vi "Trio - Connect.vi"(9 "TrioData In":T1 {"A Axis Parameters"."VPSPEED" format="%#_4g"; "A Axis Parameters"."AXISSTATUS" format="%#_4g"; "A Axis Parameters"."FE" format="%#_4g"; "A Axis Parameters"."MPOS" format="%#_4g"; "A Axis Parameters"."NTYPE" format="%#_4g"; "A Axis Parameters"."MTYPE" format="%#_4g"; "A Axis Parameters"."RS_LIMIT" format="%#_4g"; "A Axis Parameters"."FS_LIMIT" format="%#_4g"; "A Axis Parameters"."FH_IN" format="%#_4g"; "A Axis Parameters"."DATUM_IN" format="%#_4g"; "A Axis Parameters"."REV_IN" format="%#_4g"; "A Axis Parameters"."FWD_IN" format="%#_4g"; "A Axis Parameters"."REP_DIST" format="%#_4g"; "A Axis Parameters"."SERVO" format="%#_4g"; "A Axis Parameters"."DAC" format="%#_4g"; "A Axis Parameters"."FE_LIMIT" format="%#_4g"; "A Axis Parameters"."JOGSPEED" format="%#_4g"; "A Axis Parameters"."CREEP" format="%#_4g"; "A Axis Parameters"."DECEL" format="%#_4g"; "A Axis Parameters"."ACCEL" format="%#_4g"; "A Axis Parameters"."SPEED" format="%#_4g"; "A Axis Parameters"."UNITS" format="%#_4g"; "A Axis Parameters"."VFF_GAIN" format="%#_4g"; "A Axis Parameters"."0V_GAIN" format="%#_4g"; "A Axis Parameters"."D_GAIN" format="%#_4g"; "A Axis Parameters"."I_GAIN" format="%#_4g"; "A Axis Parameters"."P_GAIN" format="%#_4g"; "A Axis Parameters"."ATYPE" format="%#_4g"; "X Axis Parameters"."VPSPEED" format="%#_4g"; "X Axis Parameters"."AXISSTATUS" format="%#_4g"; "X Axis Parameters"."FE" format="%#_4g"; "X Axis Parameters"."MPOS" format="%#_4g"; "X Axis Parameters"."NTYPE" format="%#_4g"; "X Axis Parameters"."MTYPE" format="%#_4g"; "X Axis Parameters"."RS_LIMIT" format="%#_4g"; "X Axis Parameters"."FS_LIMIT" format="%#_4g"; "X Axis Parameters"."FH_IN" format="%#_4g"; "X Axis Parameters"."DATUM_IN" format="%#_4g"; "X Axis Parameters"."REV_IN" format="%#_4g"; "X Axis Parameters"."FWD_IN" format="%#_4g"; "X Axis Parameters"."REP_DIST" format="%#_4g"; "X Axis Parameters"."SERVO" format="%#_4g"; "X Axis Parameters"."DAC" format="%#_4g"; "X Axis Parameters"."FE_LIMIT" format="%#_4g"; "X Axis Parameters"."JOGSPEED" format="%#_4g"; "X Axis Parameters"."CREEP" format="%#_4g"; "X Axis Parameters"."DECEL" format="%#_4g"; "X Axis Parameters"."ACCEL" format="%#_4g"; "X Axis Parameters"."SPEED" format="%#_4g"; "X Axis Parameters"."UNITS" format="%#_4g"; "X Axis Parameters"."VFF_GAIN" format="%#_4g"; "X Axis Parameters"."0V_GAIN" format="%#_4g"; "X Axis Parameters"."D_GAIN" format="%#_4g"; "X Axis Parameters"."I_GAIN" format="%#_4g"; "X Axis Parameters"."P_GAIN" format="%#_4g"; "X Axis Parameters"."ATYPE" format="%#_4g"}, 10 "error in (no error)":errorcluster, 11 "Trio Reference In":refnum<k7>) -> (1 "TrioData Out":T1 {"A Axis Parameters"."VPSPEED" format="%#_4g"; "A Axis Parameters"."AXISSTATUS" format="%#_4g"; "A Axis Parameters"."FE" format="%#_4g"; "A Axis Parameters"."MPOS" format="%#_4g"; "A Axis Parameters"."NTYPE" format="%#_4g"; "A Axis Parameters"."MTYPE" format="%#_4g"; "A Axis Parameters"."RS_LIMIT" format="%#_4g"; "A Axis Parameters"."FS_LIMIT" format="%#_4g"; "A Axis Parameters"."FH_IN" format="%#_4g"; "A Axis Parameters"."DATUM_IN" format="%#_4g"; "A Axis Parameters"."REV_IN" format="%#_4g"; "A Axis Parameters"."FWD_IN" format="%#_4g"; "A Axis Parameters"."REP_DIST" format="%#_4g"; "A Axis Parameters"."SERVO" format="%#_4g"; "A Axis Parameters"."DAC" format="%#_4g"; "A Axis Parameters"."FE_LIMIT" format="%#_4g"; "A Axis Parameters"."JOGSPEED" format="%#_4g"; "A Axis Parameters"."CREEP" format="%#_4g"; "A Axis Parameters"."DECEL" format="%#_4g"; "A Axis Parameters"."ACCEL" format="%#_4g"; "A Axis Parameters"."SPEED" format="%#_4g"; "A Axis Parameters"."UNITS" format="%#_4g"; "A Axis Parameters"."VFF_GAIN" format="%#_4g"; "A Axis Parameters"."0V_GAIN" format="%#_4g"; "A Axis Parameters"."D_GAIN" format="%#_4g"; "A Axis Parameters"."I_GAIN" format="%#_4g"; "A Axis Parameters"."P_GAIN" format="%#_4g"; "A Axis Parameters"."ATYPE" format="%#_4g"; "X Axis Parameters"."VPSPEED" format="%#_4g"; "X Axis Parameters"."AXISSTATUS" format="%#_4g"; "X Axis Parameters"."FE" format="%#_4g"; "X Axis Parameters"."MPOS" format="%#_4g"; "X Axis Parameters"."NTYPE" format="%#_4g"; "X Axis Parameters"."MTYPE" format="%#_4g"; "X Axis Parameters"."RS_LIMIT" format="%#_4g"; "X Axis Parameters"."FS_LIMIT" format="%#_4g"; "X Axis Parameters"."FH_IN" format="%#_4g"; "X Axis Parameters"."DATUM_IN" format="%#_4g"; "X Axis Parameters"."REV_IN" format="%#_4g"; "X Axis Parameters"."FWD_IN" format="%#_4g"; "X Axis Parameters"."REP_DIST" format="%#_4g"; "X Axis Parameters"."SERVO" format="%#_4g"; "X Axis Parameters"."DAC" format="%#_4g"; "X Axis Parameters"."FE_LIMIT" format="%#_4g"; "X Axis Parameters"."JOGSPEED" format="%#_4g"; "X Axis Parameters"."CREEP" format="%#_4g"; "X Axis Parameters"."DECEL" format="%#_4g"; "X Axis Parameters"."ACCEL" format="%#_4g"; "X Axis Parameters"."SPEED" format="%#_4g"; "X Axis Parameters"."UNITS" format="%#_4g"; "X Axis Parameters"."VFF_GAIN" format="%#_4g"; "X Axis Parameters"."0V_GAIN" format="%#_4g"; "X Axis Parameters"."D_GAIN" format="%#_4g"; "X Axis Parameters"."I_GAIN" format="%#_4g"; "X Axis Parameters"."P_GAIN" format="%#_4g"; "X Axis Parameters"."ATYPE" format="%#_4g"}, 2 "error out":errorcluster, 3 "Trio Reference Out":refnum<k7>)   [LabVIEW 2020, in "TrioMotion Controller.lvlib"]
uses:
  TrioMotion Controller.lvlib
  TrioData.ctl
  Connection Type.ctl
  Axis Parameters.ctl
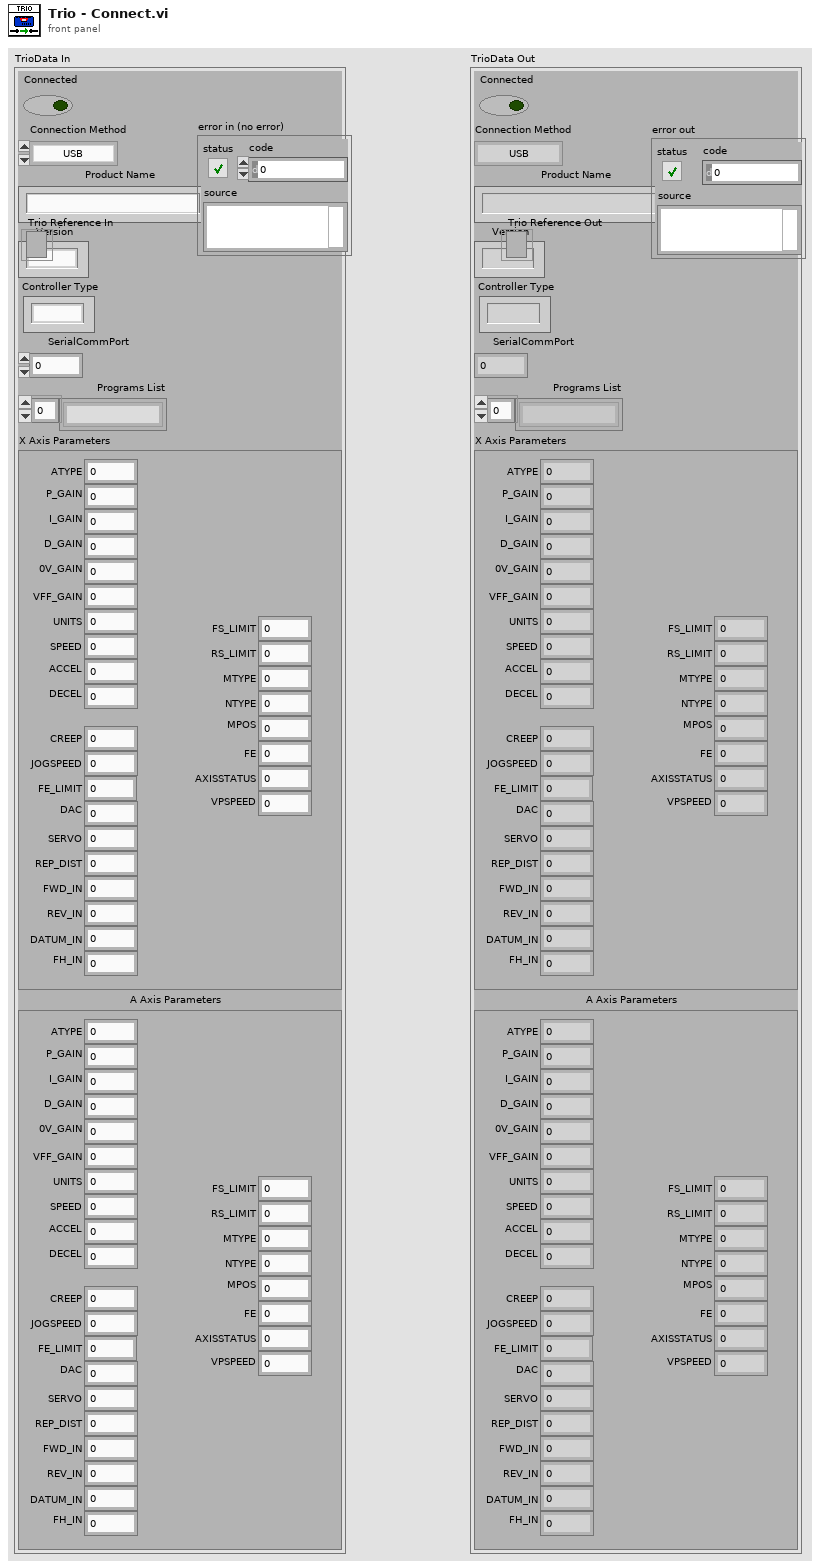
[diagram p1: front panel]
types:
  T1 = typedef "TrioMotion Controller.lvlib/TrioData.ctl" = cluster{"Connected":bool, "Connection Method":T2, "Product Name":string, " Version":string, "Controller Type":string, "SerialCommPort":fxp<+,3,3>, "Programs List":string[], "X Axis Parameters":T3, "A Axis Parameters":T3}
  T2 = typedef "TrioMotion Controller.lvlib/Connection Type.ctl" = enum16{"USB", "Serial", "Ethernet", "PCI", "Path", "No connection"}
  T3 = typedef "TrioMotion Controller.lvlib/Axis Parameters.ctl" = cluster{"ATYPE":dbl, "P_GAIN":dbl, "I_GAIN":dbl, "D_GAIN":dbl, "0V_GAIN":dbl, "VFF_GAIN":dbl, "UNITS":dbl, "SPEED":dbl, "ACCEL":dbl, "DECEL":dbl, "CREEP":dbl, "JOGSPEED":dbl, "FE_LIMIT":dbl, "DAC":dbl, "SERVO":dbl, "REP_DIST":dbl, "FWD_IN":dbl, "REV_IN":dbl, "DATUM_IN":dbl, "FH_IN":dbl, "FS_LIMIT":dbl, "RS_LIMIT":dbl, "MTYPE":dbl, "NTYPE":dbl, "MPOS":dbl, "FE":dbl, "AXISSTATUS":dbl, "VPSPEED":dbl}
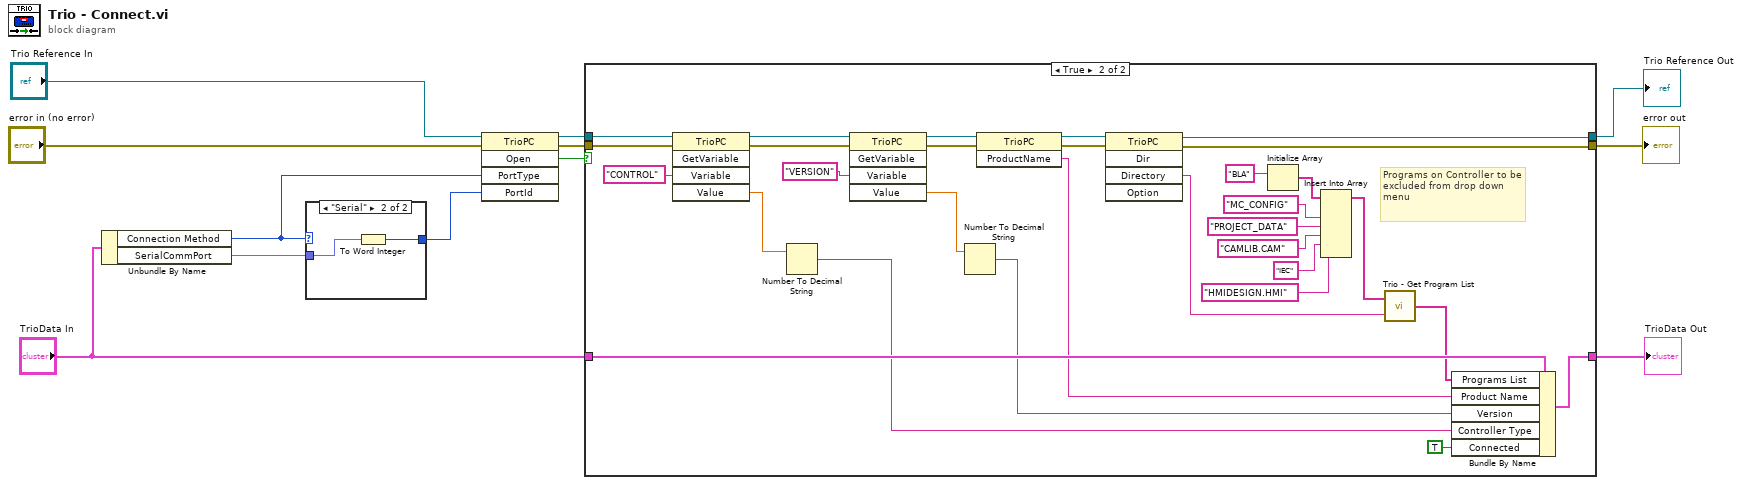
[diagram p0: block diagram]
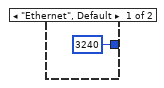
[diagram p2: hidden frame]
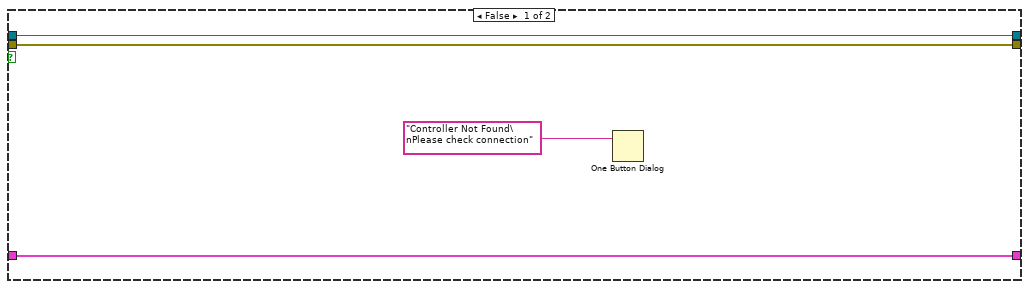
[diagram p3: hidden frame]
diagram:
  n1 = Unbundle By Name("TrioData In") -> ("Connection Method"=w1:T2, "SerialCommPort"=w3:fxp<+,3,3>)
  n2 = case shown="\"Serial\"" w1 {
    tunnel: [i16 3240 ("PortId") w14] -> w2
    tunnel: w3 -> [_ w15]
    frame "Ethernet", Default {
    }
    frame "Serial" {
      n3 = To Word Integer(number=w15) -> (16bit integer=w14:i16)
    }
  }
  n4 = invoke class="TrioPC" method="Open"(reference="Trio Reference In", error in="error in (no error)", "PortType"=w1, "PortId"=w2) -> (reference out=w4:refnum<k7>, error out=w5:errorcluster, "Open"=w6:bool)  [unwired: 1 in, 2 out]
  n5 = case shown="True" w6 {
    tunnel: [w18 w29] -> w9
    tunnel: [w19 w30] -> w10
    tunnel: w4 -> [w19 w31]
    tunnel: w5 -> [w18 w36]
    tunnel: "TrioData In" -> [w16 w28]
    tunnel: [w16 w27] -> w7
    frame False {
      n6 = One Button Dialog(message="Controller Not Found\nPlease check connection") -> ()  [unwired: 1 in, 1 out]
    }
    frame True {
      # "Programs on Controller to be excluded from drop down menu"
      n7 = invoke class="TrioPC" method="GetVariable"(reference=w31, error in=w36, "Variable"="CONTROL") -> (reference out=w38:refnum<k7>, error out=w37:errorcluster, "Value"=w41:dbl)  [unwired: 2 in, 2 out]
      n8 = Number To Decimal String(number=w41) -> (decimal integer string=w21:string)  [unwired: 1 in]
      n9 = invoke class="TrioPC" method="GetVariable"(reference=w38, error in=w37, "Variable"="VERSION") -> (reference out=w34:refnum<k7>, error out=w35:errorcluster, "Value"=w40:dbl)  [unwired: 2 in, 2 out]
      n10 = Number To Decimal String(number=w40) -> (decimal integer string=w22:string)  [unwired: 1 in]
      n11 = invoke class="TrioPC" method="ProductName"(reference=w34, error in=w35) -> (reference out=w33:refnum<k7>, error out=w32:errorcluster, "ProductName"=w23:string)  [unwired: 1 in]
      n12 = invoke class="TrioPC" method="Dir"(reference=w33, error in=w32) -> (reference out=w30:refnum<k7>, error out=w29:errorcluster, "Directory"=w25:string)  [unwired: 3 in, 2 out]
      n13 = Initialize Array("BLA" ("element")) -> (w49:string[])  [unwired: 1 in]
      n14 = Insert Into Array(array=w49, new element #1="MC_CONFIG" ("element"), new element #2="PROJECT_DATA" ("element"), new element #3="CAMLIB.CAM" ("element"), new element #4="IEC" ("element"), new element #5="HMIDESIGN.HMI") -> (w26:string[])  [unwired: 1 in]
      n15 = call "Trio - Get Program List.vi"("Controller Directory"=w25, "Exclusion List"=w26) -> ("Programs List"=w24:string[])
      n16 = Bundle By Name(cluster=w28, "Programs List"=w24, "Product Name"=w23, "Version"=w22, "Controller Type"=w21, "Connected"=TRUE) -> (w27:T1)
    }
  }
  "TrioData Out" <- w7
  "error out" <- w9
  "Trio Reference Out" <- w10
